vi "Generate.vi"() -> ()   [LabVIEW 2018, in "Scripts.lvlib"]
uses:
  Scripts.lvlib
  <vilib>/Field R&D Services/Labricator/Toolkit/Type Definitions/Help Root Folder Names.ctl
  <vilib>/Field R&D Services/Labricator/Toolkit/Field_RnD_Services_Labricator_Toolkit.lvlib
panel:
  in  "Options":T2={"Generate"={"HTML?"=TRUE, "Index?"=TRUE, "ToC?"=TRUE}, "Included Scopes"={"Community"=TRUE, "Private"=FALSE, "Protected"=TRUE, "Public"=TRUE}, "Root Folder Names"={"HTML"="pages", "Images"="images", "Scripts"="scripts", "Styles"="styles"}}
  # "Overview: Generates the HTML help documentation for the Toolkit library VIs\nRequirements: LabVIEW 2016 or newer, Labricator Development Kit\nInstructions: Run this VI.\n\nThis VI creates HTML files based on the descriptions for Controls, Classes, Indicators, Libraries, and VIs."
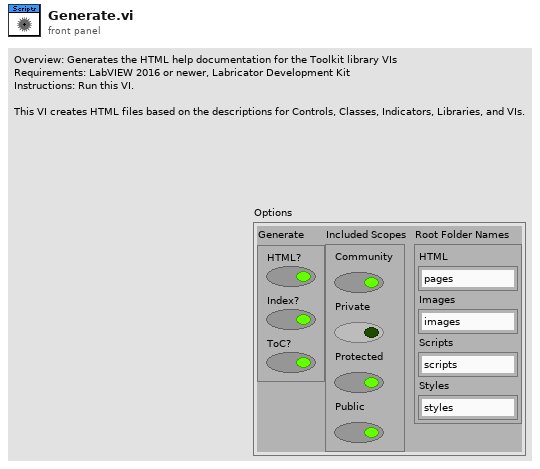
[diagram p1: front panel]
types:
  T1 = typedef "Field_RnD_Services_Labricator_Toolkit.lvlib/Help Root Folder Names.ctl" = cluster{"HTML":string, "Images":string, "Scripts":string, "Styles":string}
  T2 = cluster{"Generate":cluster{"HTML?":bool, "Index?":bool, "ToC?":bool}, "Included Scopes":cluster{"Community":bool, "Private":bool, "Protected":bool, "Public":bool}, "Root Folder Names":T1}
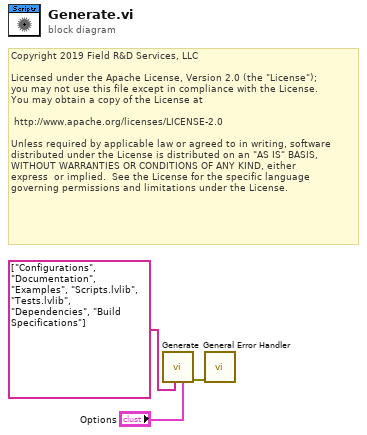
[diagram p0: block diagram]
diagram:
  # "Copyright 2019 Field R&D Services, LLC\n\nLicensed under the Apache License, Version 2.0 (the \"License\");\nyou may not use this file except in compliance with the License.\nYou may obtain a copy of the License at\n\n\thttp://www.apache.org/licenses/LICENSE-2.0\n\nUnless required by applicable law or agreed to in writing, software\ndistributed under the License is distributed on an \"AS IS\" BASIS,\nWITHOUT WARRANTIES OR CONDITIONS OF ANY KIND, either \nexpress  or implied.  See the License for the specific language \ngoverning permissions and limitations under the License."
  n1 = call <vilib>:"Generate.vi"("Options"="Options", "Excluded Project Items"=string[] ["Configurations", "Documentation", "Examples", "Scripts.lvlib", "Tests.lvlib", "Dependencies", "Build Specifications"]) -> ("Error Out"=w3:errorcluster)  [unwired: 8 in, 1 out]
  n2 = call <vilib>:"General Error Handler.vi"("error in (no error)"=w3) -> ()  [unwired: 10 in, 5 out]
